vi "Write Function Name.vi"(10 "Function Name":string, 11 "Find Compatible Hardware for Function Msg in":refnum<class "Find Compatible Hardware for Function Msg.lvclass">) -> (3 "Find Compatible Hardware for Function Msg out":refnum<class "Find Compatible Hardware for Function Msg.lvclass">)   [LabVIEW 2016, in "Controller Actor.lvlib" / "Find Compatible Hardware for Function Msg.lvclass"]
uses:
  <userlib>/Common Components/Controller/Messages/Find Compatible Hardware for Function Msg/Find Compatible Hardware for Function Msg.lvclass
  <userlib>/Common Components/Controller/Messages/Find Compatible Hardware for Function Msg/Find Compatible Hardware for Function Msg.lvclass/Find Compatible Hardware for Function Msg.ctl
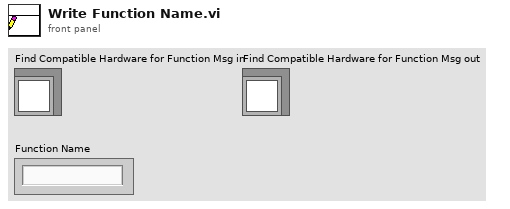
[diagram p1: front panel]
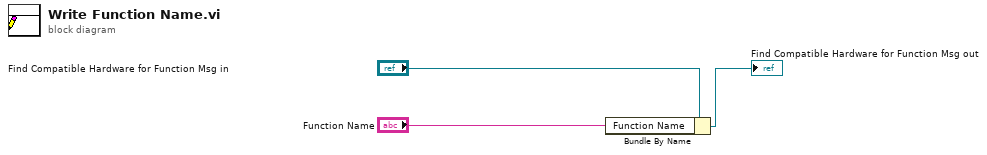
[diagram p0: block diagram]
diagram:
  n1 = Bundle By Name(cluster="Find Compatible Hardware for Function Msg in", "Function Name"="Function Name") -> (→"Find Compatible Hardware for Function Msg out":refnum<class "Find Compatible Hardware for Function Msg.lvclass">)
